vi "Configuration Parse.vi"(8 "error in":errorcluster, 11 "UI Controls":T5={"measurement configuration"={"Automation Test"=FALSE, "Power sequencing file path"="", "SMU name"="", "SMU channel"="0", "Compression_Expected DUT Gain (dB)"=0.0, "Compression_Max Linear Range (dBm)"=0.0, "Compression_Compression Point (dB)"=0.0, "Compression_Target Pin (dBm)"=1.0, "Compression_RFSG Frequency Start (Hz)"=0.0, "Compression_RFSG Frequency Stop (Hz)"=0.0, "Compression_RFSG Number of Frequency Step"=0, "Compression_RFSG Power Start (dBm)"=0.0, "Compression_RFSG Power Stop(dBm)"=0.0, "Compression_RFSG Power Step Size (dB)"=0.0, "Compression_RBW (Hz)"=0.0}, "measurement results"={"Status"="", "per Freq Plot Names"=[], "Linear Gain vs Freq"=[], "OPxdB vs Freq"=[], "Pout@Pin vs Freq"=[], "Gain@Pin vs Freq"=[], "PAE@Pin vs Freq"=[], "Pout vs Pin per Freq"=[], "Gain vs Pin per Freq"=[], "PAE vs Pin per Freq"=[], "Pout@Pin (Mean)"=0.0, "Gain@Pin (Mean)"=0.0, "PAE@Pin (Mean)"=0.0, "Linear Gain (Mean)"=0.0, "OPxdB (Mean)"=0.0}} {"measurement configuration"."Compression_Target Pin (dBm)" format="%#pdBm"}) -> (0 "error out":errorcluster, 3 "Test Configuration":T2={"Expected DUT Gain (dB)"=0.0, "Max Linear Range (dBm)"=0.0, "Compression Point (dB)"=0.0, "Pout at Pin (dBm)"=1.0, "RFSG Frequency Start (Hz)"=0.0, "RFSG Frequency Stop (Hz)"=0.0, "RFSG Number of Frequency Step"=0, "Power Start (dBm)"=0.0, "Power Stop(dBm)"=0.0, "Power Step Size (dB)"=0.0, "RBW (Hz)"=0.0} {"Pout at Pin (dBm)" format="%#pdBm"; "RFSG Frequency Stop (Hz)" format="%#_6p"; "Power Start (dBm)" format="%#_6p"; "Power Stop(dBm)" format="%#_6p"; "RFSG Frequency Start (Hz)" format="%#_6p"; "Expected DUT Gain (dB)" step=1.0 format="%#_6p"}, 5 "SMU Settings":T1={"SMU Name"="PXI1Slot15", "SMU Channel"="2"})   [LabVIEW 2023, in "FPT Framework.lvclass"]
uses:
  FPT Framework.lvclass
  Measurement Configuration.ctl
  Measurement Results.ctl
  Measurement/Controls/Test Config - Compression.ctl
  Measurement/Controls/SMU Config - Compression.ctl
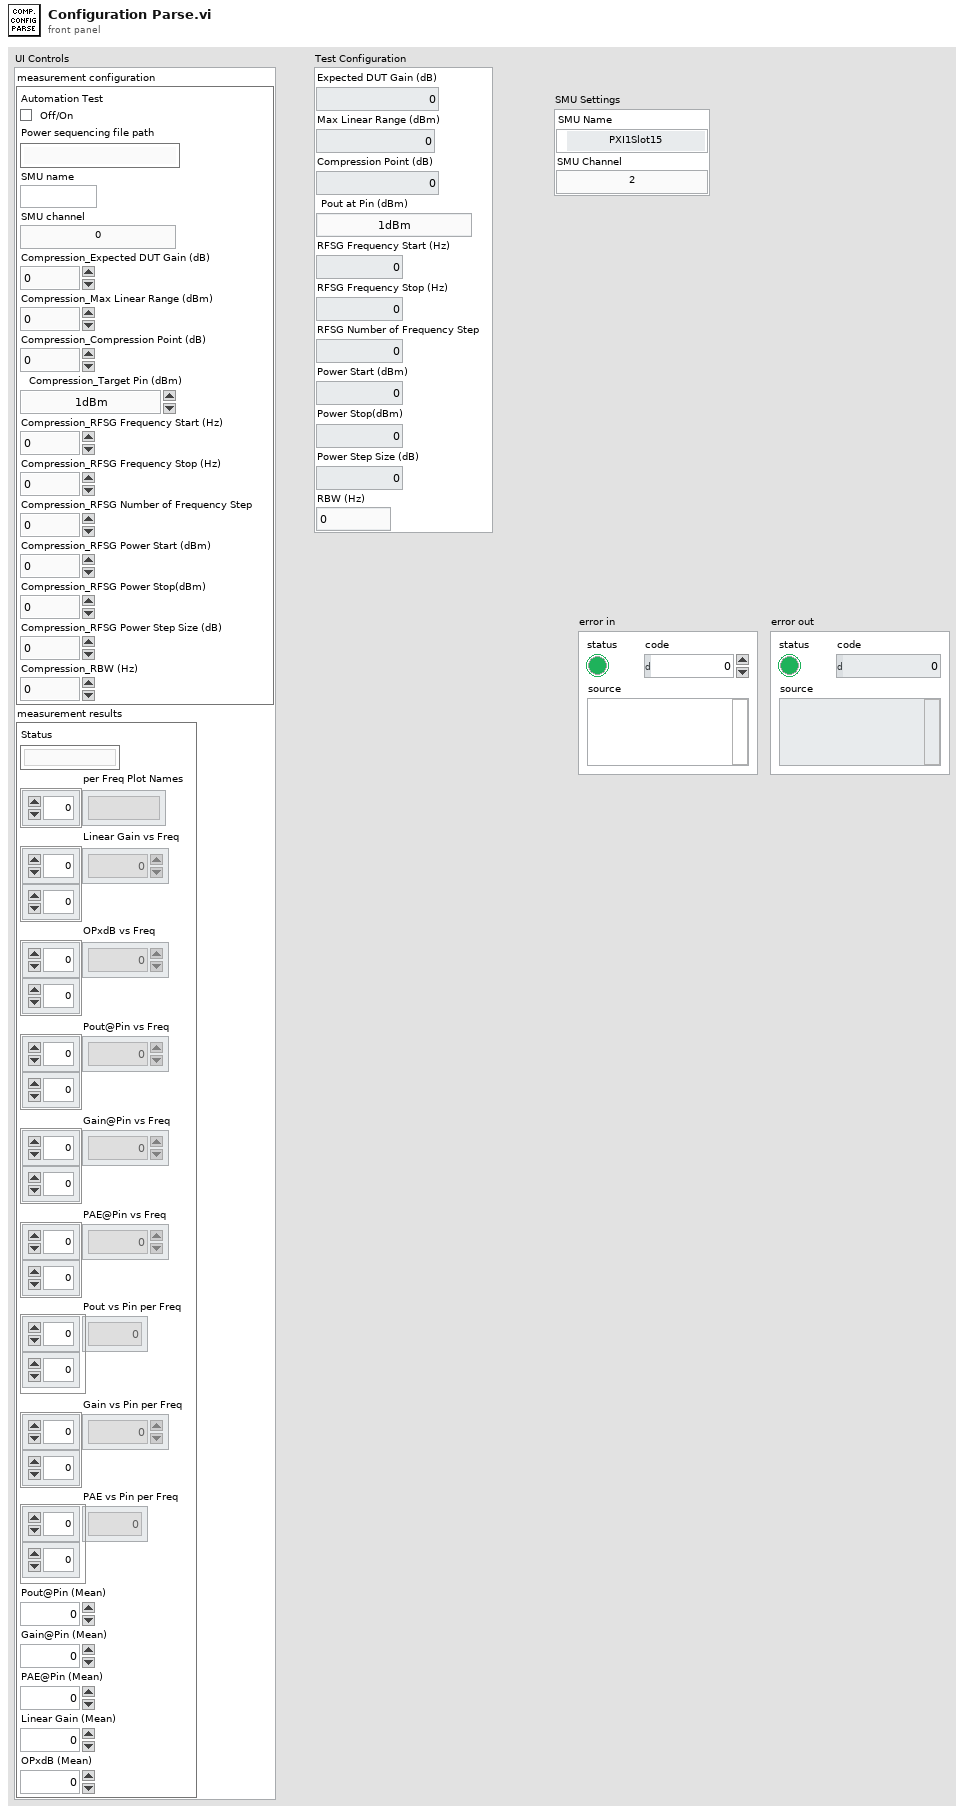
[diagram p1: front panel]
types:
  T1 = typedef "SMU Config - Compression.ctl" = cluster{"SMU Name":refnum<k15>, "SMU Channel":string}
  T2 = typedef "Test Config - Compression.ctl" = cluster{"Expected DUT Gain (dB)":dbl, "Max Linear Range (dBm)":dbl, "Compression Point (dB)":dbl, "Pout at Pin (dBm)":dbl, "RFSG Frequency Start (Hz)":dbl, "RFSG Frequency Stop (Hz)":dbl, "RFSG Number of Frequency Step":i32, "Power Start (dBm)":dbl, "Power Stop(dBm)":dbl, "Power Step Size (dB)":dbl, "RBW (Hz)":dbl}
  T3 = typedef "FPT Framework.lvclass/Measurement Configuration.ctl" = cluster{"Automation Test":bool, "Power sequencing file path":string, "SMU name":string, "SMU channel":string, "Compression_Expected DUT Gain (dB)":dbl, "Compression_Max Linear Range (dBm)":dbl, "Compression_Compression Point (dB)":dbl, "Compression_Target Pin (dBm)":dbl, "Compression_RFSG Frequency Start (Hz)":dbl, "Compression_RFSG Frequency Stop (Hz)":dbl, "Compression_RFSG Number of Frequency Step":i32, "Compression_RFSG Power Start (dBm)":dbl, "Compression_RFSG Power Stop(dBm)":dbl, "Compression_RFSG Power Step Size (dB)":dbl, "Compression_RBW (Hz)":dbl}
  T4 = typedef "FPT Framework.lvclass/Measurement Results.ctl" = cluster{"Status":string, "per Freq Plot Names":string[], "Linear Gain vs Freq":dbl[][], "OPxdB vs Freq":dbl[][], "Pout@Pin vs Freq":dbl[][], "Gain@Pin vs Freq":dbl[][], "PAE@Pin vs Freq":dbl[][], "Pout vs Pin per Freq":dbl[][], "Gain vs Pin per Freq":dbl[][], "PAE vs Pin per Freq":dbl[][], "Pout@Pin (Mean)":dbl, "Gain@Pin (Mean)":dbl, "PAE@Pin (Mean)":dbl, "Linear Gain (Mean)":dbl, "OPxdB (Mean)":dbl}
  T5 = cluster{"measurement configuration":T3, "measurement results":T4}
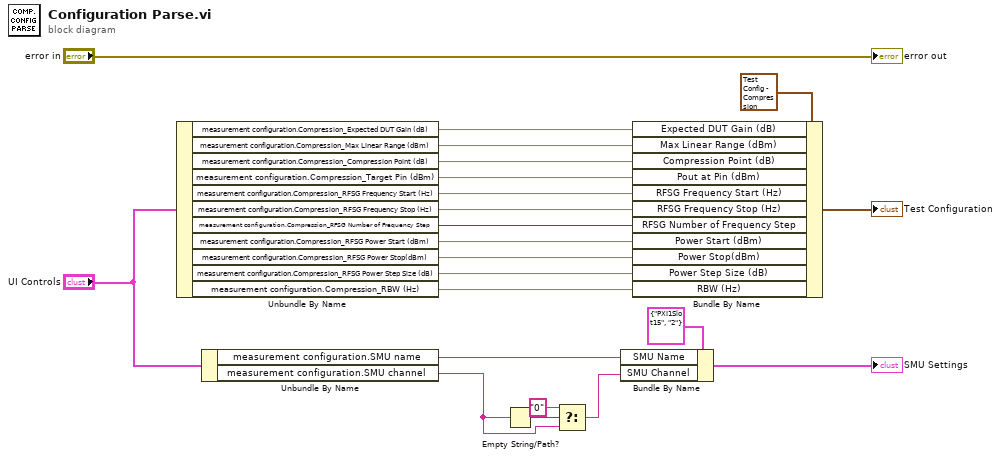
[diagram p0: block diagram]
diagram:
  n1 = Unbundle By Name("UI Controls") -> ("measurement configuration.Compression_Expected DUT Gain (dB)"=w13:dbl, "measurement configuration.Compression_Max Linear Range (dBm)"=w14:dbl, "measurement configuration.Compression_Compression Point (dB)"=w15:dbl, "measurement configuration.Compression_Target Pin (dBm)"=w5:dbl, "measurement configuration.Compression_RFSG Frequency Start (Hz)"=w16:dbl, "measurement configuration.Compression_RFSG Frequency Stop (Hz)"=w17:dbl, "measurement configuration.Compression_RFSG Number of Frequency Step"=w18:i32, "measurement configuration.Compression_RFSG Power Start (dBm)"=w19:dbl, "measurement configuration.Compression_RFSG Power Stop(dBm)"=w20:dbl, "measurement configuration.Compression_RFSG Power Step Size (dB)"=w21:dbl, "measurement configuration.Compression_RBW (Hz)"=w22:dbl)
  n2 = Unbundle By Name("UI Controls") -> ("measurement configuration.SMU name"=w6:string, "measurement configuration.SMU channel"=w2:string)
  n3 = Empty String/Path?(string/path=w2) -> (empty?=w4:bool)
  n4 = Select(t="0", s=w4, f=w2) -> (s? t:f=w3:string)
  n5 = Bundle By Name(cluster=T1 {"SMU Name"="PXI1Slot15", "SMU Channel"="2"} ("SMU Settings"), "SMU Name"=w6, "SMU Channel"=w3) -> (→"SMU Settings":T1)
  n6 = Bundle By Name(cluster=T2 {"Expected DUT Gain (dB)"=0.0, "Max Linear Range (dBm)"=0.0, "Compression Point (dB)"=0.0, "Pout at Pin (dBm)"=1.0, "RFSG Frequency Start (Hz)"=0.0, "RFSG Frequency Stop (Hz)"=0.0, "RFSG Number of Frequency Step"=0, "Power Start (dBm)"=0.0, "Power Stop(dBm)"=0.0, "Power Step Size (dB)"=0.0, "RBW (Hz)"=0.0} ("Test Configuration"), "Expected DUT Gain (dB)"=w13, "Max Linear Range (dBm)"=w14, "Compression Point (dB)"=w15, "Pout at Pin (dBm)"=w5, "RFSG Frequency Start (Hz)"=w16, "RFSG Frequency Stop (Hz)"=w17, "RFSG Number of Frequency Step"=w18, "Power Start (dBm)"=w19, "Power Stop(dBm)"=w20, "Power Step Size (dB)"=w21, "RBW (Hz)"=w22) -> (→"Test Configuration":T2)
  "error out" <- "error in"
